vi "QSPARK_setRepRate.vi"(10 "Rep Rate":u16(ring)=1 items=["20 Hz"=1, "10 Hz"=2, "5 Hz"=4, "4 Hz"=5, "2 Hz"=10, "1 Hz"=20], 11 "client handle":T1) -> (3 "client handle out":T1)   [LabVIEW 2024]
uses:
  <vilib>/httpClient/LabVIEWHTTPClient.lvlib
  <vilib>/httpClient/ClientHandle.ctl
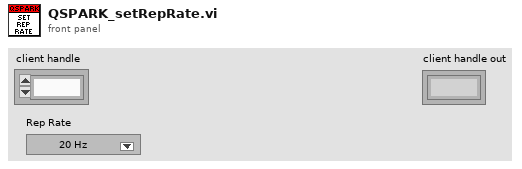
[diagram p1: front panel]
types:
  T1 = typedef "LabVIEWHTTPClient.lvlib/ClientHandle.ctl" = refnum<k1>
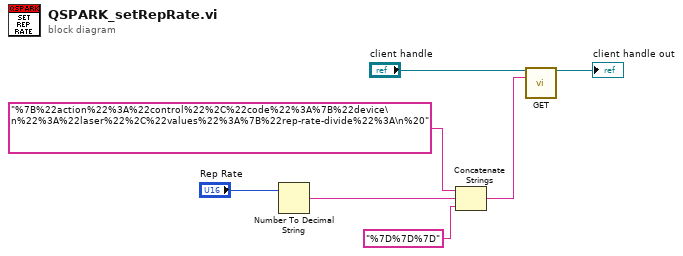
[diagram p0: block diagram]
diagram:
  n1 = Number To Decimal String(number="Rep Rate") -> (decimal integer string=w5:string)  [unwired: 1 in]
  n2 = Concatenate Strings("%7B%22action%22%3A%22control%22%2C%22code%22%3A%7B%22device\n%22%3A%22laser%22%2C%22values%22%3A%7B%22rep-rate-divide%22%3A\n%20", w5, "%7D%7D%7D" ("string")) -> (w2:string)
  n3 = call <vilib>:"GET.vi"("client handle"="client handle", "url"=w2) -> ("client handle out"=→"client handle out":T1)  [unwired: 10 in, 3 out]
